vi "Chroma 1905x Series Get IR Configuration.vi"(0 "inst handle in":refnum<visa-resource-name>, 3 "Step Number":dbl=1.0 min=1.0 max=25.0 step=1.0, 5 "error in":T1) -> (9 "Test Time":string, 11 "Channels High":string, 12 "Voltage Level":string, 13 "Channels Low":string, 14 "inst handle out":refnum<visa-resource-name>, 15 "Hi Limit":string, 16 "Low Limit":string, 18 "Ramp Time":string, 19 "error out":T1)   [LabVIEW 2025]
doc: "Contact Chroma\nTEL: +886-2-2298-3855 \nTEL: +886-3-397-5788 \nFAX: +886-2-2298-3596\nFAX: +886-3-327-4703 \nURL: http://www.chromaate.com \nE-mail: chroma@chroma.com.tw"
uses:
  <instrlib>/Chroma 19052/Chroma 19052.lvlib
panel:
  # "Get Configuration Screen"
  # "Get IR Configuration"
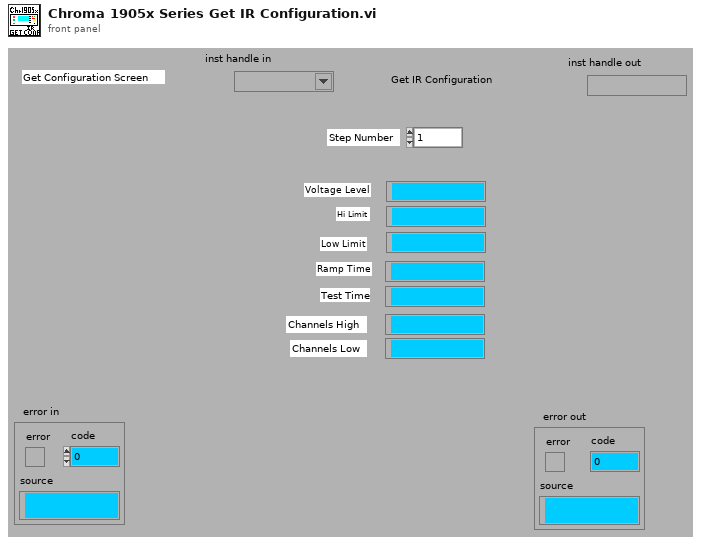
[diagram p1: front panel]
types:
  T1 = cluster{"error":bool, "code":i8, "source":string}
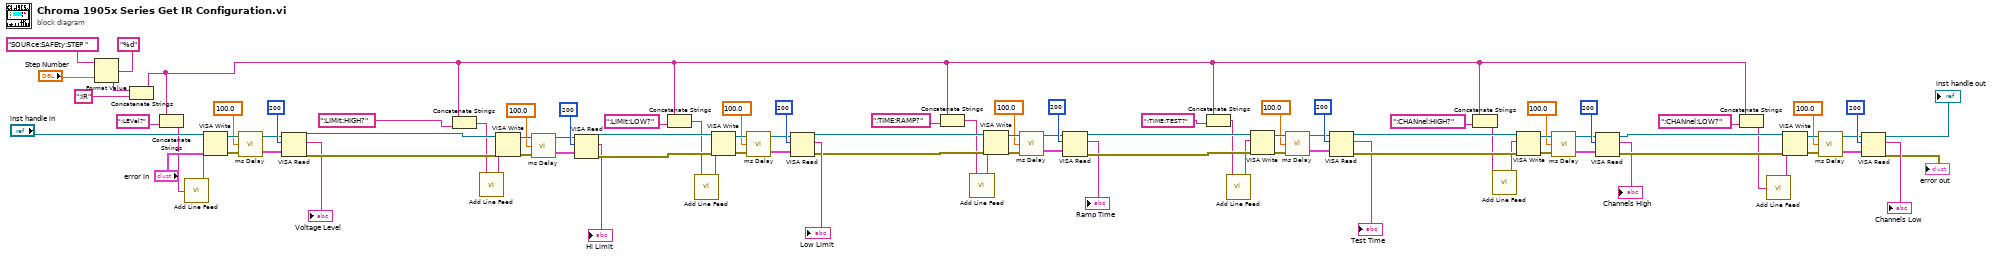
[diagram p0: block diagram]
diagram:
  n1 = Format Value(string ("")="SOURce:SAFEty:STEP ", format string="%d", value (0)="Step Number") -> (output string=w23:string)
  n2 = Concatenate Strings(w23, ":IR") -> (w20:string)
  n3 = Concatenate Strings(w20, ":LEVel?") -> (w2:string)
  n4 = call <instrlib>:"Add Line Feed.vi"("Cmdstring"=w2) -> ("Concatenated String"=w1:string)
  n5 = VISA Write(VISA resource name="inst handle in", write buffer=w1, error in (no error)="error in") -> (VISA resource name out=w84:refnum<visa-resource-name>, error out=w87:errorcluster)  [unwired: 1 out]
  n6 = call <instrlib>:"ms Delay.vi"("error in"=w87, "Time Delay S"=100.0, "inst handle in"=w84) -> ("error out"=w86:T1, "inst handle Out"=w85:refnum<visa-resource-name>)
  n7 = VISA Read(VISA resource name=w85, byte count=u32 200 ("byte count (0)"), error in (no error)=w86) -> (VISA resource name out=w74:refnum<visa-resource-name>, read buffer=→"Voltage Level":string, error out=w75:errorcluster)  [unwired: 1 out]
  n8 = Concatenate Strings(w20, ":LIMit:HIGH?") -> (w4:string)
  n9 = call <instrlib>:"Add Line Feed.vi"("Cmdstring"=w4) -> ("Concatenated String"=w3:string)
  n10 = VISA Write(VISA resource name=w74, write buffer=w3, error in (no error)=w75) -> (VISA resource name out=w77:refnum<visa-resource-name>, error out=w80:errorcluster)  [unwired: 1 out]
  n11 = call <instrlib>:"ms Delay.vi"("error in"=w80, "Time Delay S"=100.0, "inst handle in"=w77) -> ("error out"=w79:T1, "inst handle Out"=w78:refnum<visa-resource-name>)
  n12 = VISA Read(VISA resource name=w78, byte count=u32 200 ("byte count (0)"), error in (no error)=w79) -> (VISA resource name out=w65:refnum<visa-resource-name>, read buffer=→"Hi Limit":string, error out=w66:errorcluster)  [unwired: 1 out]
  n13 = Concatenate Strings(w20, ":LIMit:LOW?") -> (w6:string)
  n14 = call <instrlib>:"Add Line Feed.vi"("Cmdstring"=w6) -> ("Concatenated String"=w5:string)
  n15 = VISA Write(VISA resource name=w65, write buffer=w5, error in (no error)=w66) -> (VISA resource name out=w68:refnum<visa-resource-name>, error out=w71:errorcluster)  [unwired: 1 out]
  n16 = call <instrlib>:"ms Delay.vi"("error in"=w71, "Time Delay S"=100.0, "inst handle in"=w68) -> ("error out"=w70:T1, "inst handle Out"=w69:refnum<visa-resource-name>)
  n17 = VISA Read(VISA resource name=w69, byte count=u32 200 ("byte count (0)"), error in (no error)=w70) -> (VISA resource name out=w19:refnum<visa-resource-name>, read buffer=→"Low Limit":string, error out=w18:errorcluster)  [unwired: 1 out]
  n18 = Concatenate Strings(w20, ":TIME:RAMP?") -> (w8:string)
  n19 = call <instrlib>:"Add Line Feed.vi"("Cmdstring"=w8) -> ("Concatenated String"=w7:string)
  n20 = VISA Write(VISA resource name=w19, write buffer=w7, error in (no error)=w18) -> (VISA resource name out=w56:refnum<visa-resource-name>, error out=w59:errorcluster)  [unwired: 1 out]
  n21 = call <instrlib>:"ms Delay.vi"("error in"=w59, "Time Delay S"=100.0, "inst handle in"=w56) -> ("error out"=w58:T1, "inst handle Out"=w57:refnum<visa-resource-name>)
  n22 = VISA Read(VISA resource name=w57, byte count=u32 200 ("byte count (0)"), error in (no error)=w58) -> (VISA resource name out=w31:refnum<visa-resource-name>, read buffer=→"Ramp Time":string, error out=w30:errorcluster)  [unwired: 1 out]
  n23 = Concatenate Strings(w20, ":TIME:TEST?") -> (w10:string)
  n24 = call <instrlib>:"Add Line Feed.vi"("Cmdstring"=w10) -> ("Concatenated String"=w9:string)
  n25 = VISA Write(VISA resource name=w31, write buffer=w9, error in (no error)=w30) -> (VISA resource name out=w49:refnum<visa-resource-name>, error out=w52:errorcluster)  [unwired: 1 out]
  n26 = call <instrlib>:"ms Delay.vi"("error in"=w52, "Time Delay S"=100.0, "inst handle in"=w49) -> ("error out"=w51:T1, "inst handle Out"=w50:refnum<visa-resource-name>)
  n27 = VISA Read(VISA resource name=w50, byte count=u32 200 ("byte count (0)"), error in (no error)=w51) -> (VISA resource name out=w32:refnum<visa-resource-name>, read buffer=→"Test Time":string, error out=w28:errorcluster)  [unwired: 1 out]
  n28 = Concatenate Strings(w20, ":CHANnel:HIGH?") -> (w12:string)
  n29 = call <instrlib>:"Add Line Feed.vi"("Cmdstring"=w12) -> ("Concatenated String"=w11:string)
  n30 = VISA Write(VISA resource name=w32, write buffer=w11, error in (no error)=w28) -> (VISA resource name out=w42:refnum<visa-resource-name>, error out=w45:errorcluster)  [unwired: 1 out]
  n31 = call <instrlib>:"ms Delay.vi"("error in"=w45, "Time Delay S"=100.0, "inst handle in"=w42) -> ("error out"=w44:T1, "inst handle Out"=w43:refnum<visa-resource-name>)
  n32 = VISA Read(VISA resource name=w43, byte count=u32 200 ("byte count (0)"), error in (no error)=w44) -> (VISA resource name out=w33:refnum<visa-resource-name>, read buffer=→"Channels High":string, error out=w29:errorcluster)  [unwired: 1 out]
  n33 = Concatenate Strings(w20, ":CHANnel:LOW?") -> (w14:string)
  n34 = call <instrlib>:"Add Line Feed.vi"("Cmdstring"=w14) -> ("Concatenated String"=w13:string)
  n35 = VISA Write(VISA resource name=w33, write buffer=w13, error in (no error)=w29) -> (VISA resource name out=w35:refnum<visa-resource-name>, error out=w38:errorcluster)  [unwired: 1 out]
  n36 = call <instrlib>:"ms Delay.vi"("error in"=w38, "Time Delay S"=100.0, "inst handle in"=w35) -> ("error out"=w37:T1, "inst handle Out"=w36:refnum<visa-resource-name>)
  n37 = VISA Read(VISA resource name=w36, byte count=u32 200 ("byte count (0)"), error in (no error)=w37) -> (VISA resource name out=→"inst handle out":refnum<visa-resource-name>, read buffer=→"Channels Low":string, error out=→"error out":errorcluster)  [unwired: 1 out]
